vi "Fit Circle to Find Ball.vi"(6 "Area Size Limit":dbl=1200.0 format="%#_13g", 7 "Color Mode":u16(ring)=2 items=["RGB", "HSL", "HSV", "HSI"], 8 "Hue":cluster{dbl, dbl}(knob)={65.11832883917573, 192.11731095312356} scale=0.0..255.0 scale format="%#_3g", 9 "ROI Descriptor":T3 {"Contours"."Type" items=["No Selection", "Point", "Line", "Rectangle", "Oval", "Polygon", "Freehand Region", "Annulus", "Unused2", "Unused3", "Broken Line", "Freehand Line", "Rotated Rectangle"]}, 10 "Rectangle ltrb":dbl[](array[numeric]), 11 "Color Image In":T2) -> (1 "Potential Ball":T1, 3 "Image out":T2)   [LabVIEW 2025]
doc: "Use the ROI and rectangle to process the original image further. It is masked looking almost exclusively at hue, and then the largest particle is fitted with a circle."
uses:
  <vilib>/vision/Image Controls.llb/IMAQ Image.ctl
  <vilib>/vision/Measure.llb/Edge Options.ctl
  <vilib>/vision/Measure.llb/Edge Polarity.ctl
  <vilib>/vision/NI_Vision_Development_Module.lvlib
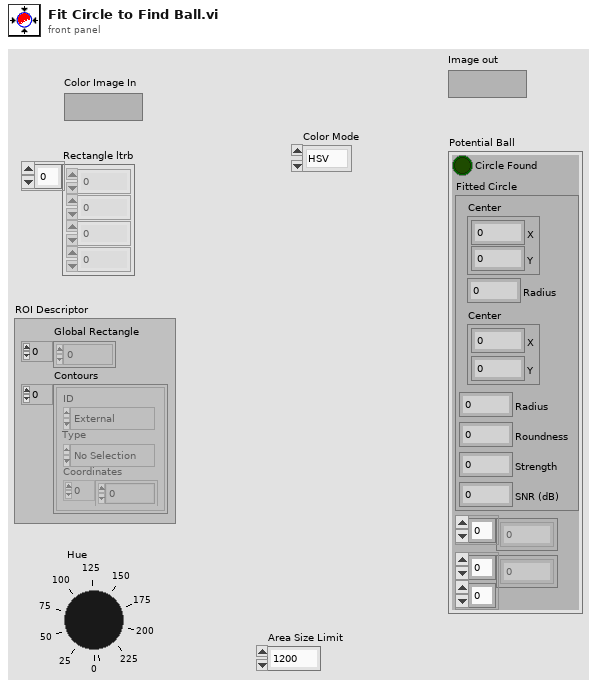
[diagram p1: front panel]
types:
  T1 = cluster{"Circle Found":bool, "Fitted Circle":cluster{"Center":cluster{"X":sgl, "Y":sgl}, "Radius":dbl, "Center":cluster{"X":sgl, "Y":sgl}, "Radius":dbl, "Roundness":dbl, "Strength":dbl, "SNR (dB)":dbl}, "Array":dbl[], "Sorted Data":dbl[][]}
  T2 = typedef "IMAQ Image.ctl" = refnum<image>
  T3 = typedef "ROI Descriptor" = cluster{"Global Rectangle":i32[], "Contours":cluster{"ID":enum32{"External", "Internal"}, "Type":u32, "Coordinates":i32[]}[]}
  T4 = typedef "Image Type" = u32
  T5 = typedef "Particle Parameters" = i32
  T6 = cluster{"Process":enum16{"Get First Edge", "Get First + Last Edge", "Get All Edges", "Get Best Edge"}, "Step Size":dbl, "Max Pixel Radius":i32}
  T7 = typedef "Edge Options.ctl" = cluster{"Edge Polarity":T8, "Kernel Size":u32, "Width":u32, "Minimum Edge Strength":sgl, "Interpolation Type":enum32{"Zero Order", "Bilinear", "Quadratic", "Cubic", "Bilinear Fixed"}, "Data Processing Method":enum32{"Average", "Median"}}
  T8 = typedef "Edge Polarity.ctl" = u32
  T9 = cluster{"Search  Direction":u32, "Edge Options":T7, "Show Search Area":bool, "Show Search Lines":bool, "Show Edges Found":bool, "Show Result":bool, "Search Area Color":u32, "Search Lines Color":u32, "Edge Locations Color":u32, "Result Color":u32, "Overlay Group Name":string}
  T10 = cluster{"Center (Pixels)":cluster{"X":sgl, "Y":sgl}, "Radius (Pixels)":dbl, "Center (Real-World)":cluster{"X":sgl, "Y":sgl}, "Radius (Real-World)":dbl, "Roundness (Real-World)":dbl, "Average Strength":dbl, "Average SNR (dB)":dbl}
  T11 = cluster{"Circle Found":bool, "Fitted Circle":cluster{"Center (Pixels)":cluster{"X":sgl, "Y":sgl}, "Radius (Pixels)":dbl, "Center (Real-World)":cluster{"X":sgl, "Y":sgl}, "Radius (Real-World)":dbl, "Roundness (Real-World)":dbl, "Average Strength":dbl, "Average SNR (dB)":dbl}, "Rectangle ltrb":dbl[], "Sorted Data":dbl[][]}
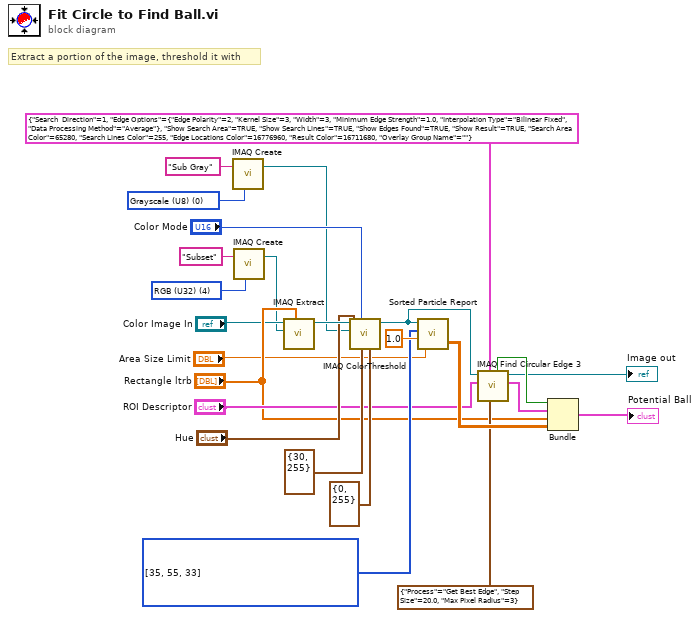
[diagram p0: block diagram]
diagram:
  w6 = T4 4 items=["Grayscale (U8)", "Grayscale (I16)", "Grayscale (SGL)", "Complex (CSG)", "RGB (U32)", "HSL (U32)", "RGB (U64)", "Grayscale (U16)"] ("Image Type")
  w8 = T4 0 items=["Grayscale (U8)", "Grayscale (I16)", "Grayscale (SGL)", "Complex (CSG)", "RGB (U32)", "HSL (U32)", "RGB (U64)", "Grayscale (U16)"] ("Image Type")
  w17 = T5[] [35, 55, 33] items=["Center of Mass X", "Center of Mass Y", "First Pixel X", "First Pixel Y", "Bounding Rect Left", "Bounding Rect Top", "Bounding Rect Right", "Bounding Rect Bottom", "Max Feret Diameter Start X", "Max Feret Diameter Start Y", "Max Feret Diameter End X", "Max Feret Diameter End Y", "Max Horiz. Segment Length Left", "Max Horiz. Segment Length Right", "Max Horiz. Segment Length Row", "-", "Bounding Rect Width", "Bounding Rect Height", "Bounding Rect Diagonal", "Perimeter", "Convex Hull Perimeter", "Holes' Perimeter", "Max Feret Diameter", "Equivalent Ellipse Major Axis", "Equivalent Ellipse Minor Axis", "Equivalent Ellipse Minor Axis (Feret)", "Equivalent Rect Long Side", "Equivalent Rect Short Side", "Equivalent Rect Diagonal", "Equivalent Rect Short Side (Feret)", "Average Horiz. Segment Length", "Average Vert. Segment Length", "Hydraulic Radius", "Waddel Disk Diameter", "-", "Area", "Holes' Area", "Particle & Holes' Area", "Convex Hull Area", "Image Area", "-", "Number of Holes", "Number of Horiz. Segments", "Number of Vert. Segments", "-", "Orientation", "Max Feret Diameter Orientation", "-", "% Area/Image Area", "% Area/(Particle & Holes' Area)", "Ratio of Equivalent Ellipse Axes", "Ratio of Equivalent Rect Sides", "-", "Elongation Factor", "Compactness Factor", "Heywood Circularity Factor", "Type Factor", "-", "Sum X", "Sum Y", "Sum XX", "Sum XY", "Sum YY", "Sum XXX", "Sum XXY", "Sum XYY", "Sum YYY", "-", "Moment of Inertia XX", "Moment of Inertia XY", "Moment of Inertia YY", "Moment of Inertia XXX", "Moment of Inertia XXY", "Moment of Inertia XYY", "Moment of Inertia YYY", "Norm. Moment of Inertia XX", "Norm. Moment of Inertia XY", "Norm. Moment of Inertia YY", "Norm. Moment of Inertia XXX", "Norm. Moment of Inertia XXY", "Norm. Moment of Inertia XYY", "Norm. Moment of Inertia YYY", "Hu Moment 1", "Hu Moment 2", "Hu Moment 3", "Hu Moment 4", "Hu Moment 5", "Hu Moment 6", "Hu Moment 7"] ("Pixel Measurements")
  # "Extract a portion of the image, threshold it with"
  n1 = call "IMAQ Create"("Image Name"="Sub Gray", "Image Type"=w8) -> ("New Image"=w3:T2)  [unwired: 3 in, 1 out]
  n2 = call "IMAQ Create"("Image Name"="Subset", "Image Type"=w6) -> ("New Image"=w2:T2)  [unwired: 3 in, 1 out]
  n3 = call "IMAQ Extract"("Optional Rectangle"="Rectangle ltrb", "Image Dst"=w2, "Image Src"="Color Image In") -> ("Image Dst Out"=w22:T2)  [unwired: 7 in, 1 out]
  n4 = call "IMAQ ColorThreshold"("Blue or Luma or Val or Inten Range"=cluster{"Lower value":i32, "Upper value":i32} {"Lower value"=0, "Upper value"=255} ("Red or Hue Range 3"), "Green or Sat Range"=cluster{"Lower value":i32, "Upper value":i32} {"Lower value"=30, "Upper value"=255} ("Red or Hue Range 3"), "Color Mode"="Color Mode", "Red or Hue Range"="Hue", "Image Dst"=w3, "Image Src"=w22) -> ("Image Dst Out"=w25:T2)  [unwired: 4 in, 1 out]
  n5 = call "Sorted Particle Report.vi"("Area Size Limit"="Area Size Limit", "Particle Count Limit"=1.0, "Pixel Measurements"=w17, "Image in"=w25) -> ("Sorted Data"=w24:dbl[][])  [unwired: 1 out]
  n6 = call "IMAQ Find Circular Edge 3"("Circle Fit Options"=T6 {"Process"=enum."Get Best Edge", "Step Size"=20.0, "Max Pixel Radius"=3}, "Options"=T9 {"Search  Direction"=1, "Edge Options"={"Edge Polarity"=2, "Kernel Size"=3, "Width"=3, "Minimum Edge Strength"=1.0, "Interpolation Type"=enum."Bilinear Fixed", "Data Processing Method"=enum."Average"}, "Show Search Area"=TRUE, "Show Search Lines"=TRUE, "Show Edges Found"=TRUE, "Show Result"=TRUE, "Search Area Color"=65280, "Search Lines Color"=255, "Edge Locations Color"=16776960, "Result Color"=16711680, "Overlay Group Name"=""}, "ROI Descriptor"="ROI Descriptor", "Image"=w25) -> ("Fitted Circle"=w21:T10, "Image Out"=→"Image out":T2, "Circle Found"=w20:bool)  [unwired: 3 in, 2 out]
  n7 = Bundle("Circle Found"=w20, "Fitted Circle"=w21, "Rectangle ltrb"="Rectangle ltrb", "Sorted Data"=w24) -> (→"Potential Ball":T11)  [unwired: 1 in]
